vi "Write Status.vi"(8 "error in (no error)":errorcluster, 10 "Dome Contents":T1, 11 "Dome in":refnum<class "Dome.lvclass">) -> (0 "error out":errorcluster, 3 "Dome out":refnum<class "Dome.lvclass">)   [LabVIEW 2018, in "Dome.lvclass"]
uses:
  Dome.lvclass
  Dome.lvclass/Dome.ctl
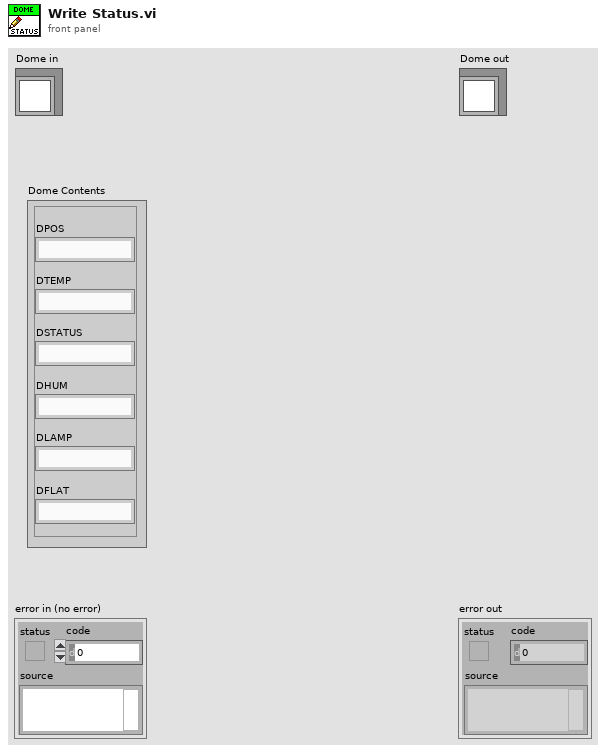
[diagram p1: front panel]
types:
  T1 = cluster{"DSTATUS":string, "DPOS":string, "DTEMP":string, "DHUM":string, "DLAMP":string, "DFLAT":string}
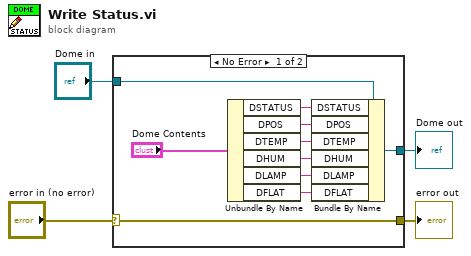
[diagram p0: block diagram]
diagram:
  n1 = case shown="No Error" "error in (no error)" {
    selector: "error in (no error)" -> [w14 w16]
    tunnel: [w14 w16] -> w3
    tunnel: [w12 w15] -> w1
    tunnel: "Dome in" -> [w13 w15]
    frame No Error {
      n2 = Unbundle By Name("Dome Contents") -> ("DSTATUS"=w5:string, "DPOS"=w6:string, "DTEMP"=w7:string, "DHUM"=w8:string, "DLAMP"=w9:string, "DFLAT"=w10:string)
      n3 = Bundle By Name(cluster=w13, "DSTATUS"=w5, "DPOS"=w6, "DTEMP"=w7, "DHUM"=w8, "DLAMP"=w9, "DFLAT"=w10) -> (w12:refnum<class "Dome.lvclass">)
    }
    frame Error {
    }
  }
  "error out" <- w3
  "Dome out" <- w1
